vi "ReadImage.vi"(10 "Draw Area Size":T1, 11 "Image path":path) -> (0 "success?":bool, 2 "Image":picture, 3 "zoom":dbl)   [LabVIEW 2024]
uses:
  <vilib>/Utility/miscctls.llb/LVBoundsTypeDef.ctl
  <vilib>/picture/picture.llb/imagedata.ctl
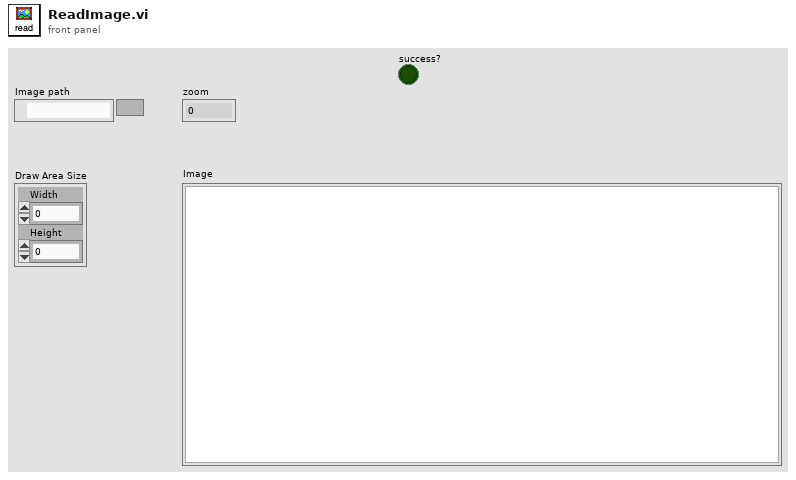
[diagram p1: front panel]
types:
  T1 = typedef "LVBoundsTypeDef.ctl" = cluster{"Width":u32, "Height":u32}
  T2 = typedef "imagedata.ctl" = cluster{"image type":i32, "image depth":i32, "image":u8[], "mask":u8[], "colors":u32[], "Rectangle":cluster{"left":i16, "top":i16, "right":i16, "bottom":i16}}
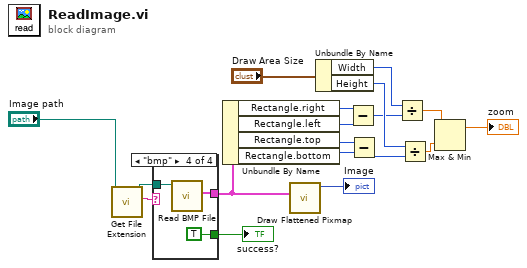
[diagram p0: block diagram]
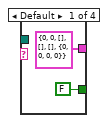
[diagram p2: hidden frame]
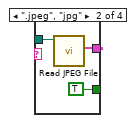
[diagram p3: hidden frame]
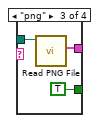
[diagram p4: hidden frame]
diagram:
  n1 = call <vilib>:"Get File Extension.vi"("file"="Image path") -> ("lowercase file extension"=w3:string, "dup file"=w4:path)  [unwired: 6 in, 3 out]
  n2 = case shown="\"bmp\"" w3 {
    tunnel: w4 -> [_ w23 w26 w29]
    tunnel: [T2 {"image type"=0, "image depth"=0, "image"=[], "mask"=[], "colors"=[], "Rectangle"={"left"=0, "top"=0, "right"=0, "bottom"=0}} ("image data") w22 w25 w28] -> w6
    tunnel: [FALSE TRUE TRUE TRUE] -> w1
    frame Default {
    }
    frame ".jpeg", "jpg" {
      n3 = call <vilib>:"Read JPEG File.vi"("path to JPEG file"=w23) -> ("image data"=w22:T2)  [unwired: 8 in, 2 out]
    }
    frame "png" {
      n4 = call <vilib>:"Read PNG File.vi"("path to PNG file"=w26) -> ("image data"=w25:T2)  [unwired: 8 in, 2 out]
    }
    frame "bmp" {
      n5 = call <vilib>:"Read BMP File.vi"("path to BMP file"=w29) -> ("image data"=w28:T2)  [unwired: 8 in, 2 out]
    }
  }
  "success?" <- w1
  n6 = Unbundle By Name(w6) -> ("Rectangle.right"=w9:i16, "Rectangle.left"=w10:i16, "Rectangle.top"=w7:i16, "Rectangle.bottom"=w8:i16)
  n7 = call <vilib>:"Draw Flattened Pixmap.vi"("image data"=w6) -> ("new picture"=→"Image":picture)  [unwired: 8 in]
  n8 = Unbundle By Name("Draw Area Size") -> ("Width"=w15:u32, "Height"=w17:u32)
  n9 = Subtract(x=w9, y=w10) -> (x-y=w16:i16)
  n10 = Subtract(x=w7, y=w8) -> (x-y=w18:i16)
  n11 = Divide(x=w15, y=w16) -> (x/y=w13:dbl)
  n12 = Divide(x=w17, y=w18) -> (x/y=w12:dbl)
  n13 = Max & Min(x=w13, y=w12) -> (max(x,y)=→"zoom":dbl)  [unwired: 1 out]
